vi "SGDA-Compute Frame Properties.vi"(8 "Pts/rep":i32, 9 "reps/frame":i32=1, 10 "Fs (Hz)":dbl, 11 "Nominal Framesize (s)":dbl=0.5) -> (1 "reps/frame":i32, 3 "pts/frame":i32)   [LabVIEW 2020]
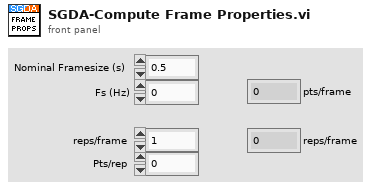
[diagram p1: front panel]
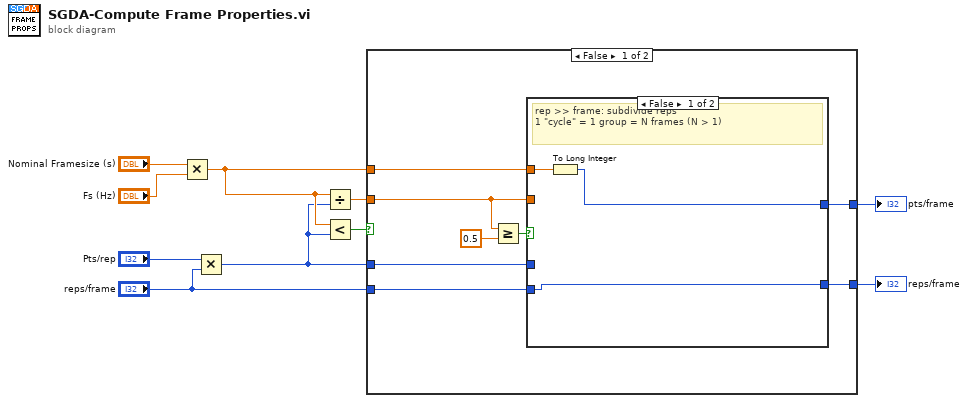
[diagram p0: block diagram]
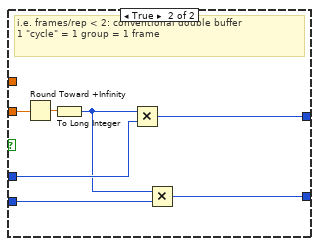
[diagram p2: hidden frame]
diagram:
  n1 = Multiply(x="Nominal Framesize (s)", y="Fs (Hz)") -> (x*y=w3:dbl)
  n2 = Multiply(x="Pts/rep", y="reps/frame") -> (x*y=w2:i32)
  n3 = Divide(x=w3, y=w2) -> (x/y=w8:dbl)
  n4 = Less?(x=w3, y=w2) -> (x < y?=w1:bool)
  n5 = case shown="False" w1 {
    tunnel: w8 -> [w18 _]
    tunnel: [w15 w30] -> w6
    tunnel: [w14 w29] -> w5
    tunnel: "reps/frame" -> [w13 w29]
    tunnel: w3 -> [w12 _]
    tunnel: w2 -> [w11 w30]
    frame False {
      n6 = Greater Or Equal?(x=w18, y=0.5) -> (x >= y?=w16:bool)
      n7 = case shown="False" w16 {
        tunnel: w18 -> [_ w27]
        tunnel: w11 -> [_ w26]
        tunnel: [w20 w25] -> w15
        tunnel: [w19 w24] -> w14
        tunnel: w13 -> [w19 w23]
        tunnel: w12 -> [w21 _]
        frame False {
          # "rep >> frame: subdivide reps\n1 \"cycle\" = 1 group = N frames (N > 1)"
          n8 = To Long Integer(number=w21) -> (32bit integer=w20:i32)
        }
        frame True {
          # "i.e. frames/rep < 2: conventional double buffer\n1 \"cycle\" = 1 group = 1 frame"
          n9 = Round Toward +Infinity(x=w27) -> (ceil(x): smallest int >= x=w28:dbl)
          n10 = To Long Integer(number=w28) -> (32bit integer=w22:i32)
          n11 = Multiply(x=w22, y=w26) -> (x*y=w25:i32)
          n12 = Multiply(x=w22, y=w23) -> (x*y=w24:i32)
        }
      }
    }
    frame True {
    }
  }
  "pts/frame" <- w6
  "reps/frame" <- w5
